vi "ActivateToggleControls (SubVI).vi"(0 "Left refnum":refnum<vi>, 1 "Current stage position [mm]":cluster{"X":dbl, "Y":dbl, "Z":dbl}, 5 "Right refnum":refnum<vi>, 7 "Forward refnum":refnum<vi>, 9 "Backward refnum":refnum<vi>, 11 "error in (no error)":errorcluster, 12 "Jog step size":T1) -> (15 "error out":errorcluster)   [LabVIEW 2016]
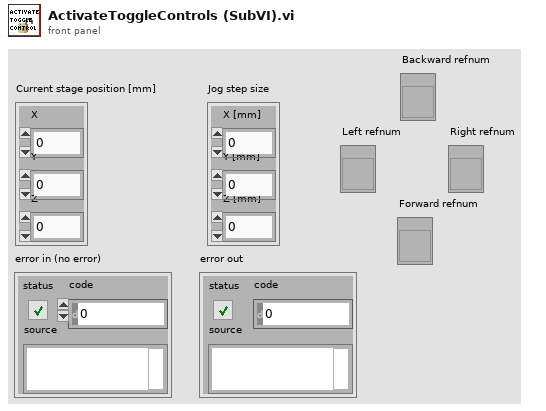
[diagram p1: front panel]
types:
  T1 = cluster{"X [mm]":dbl, "Y [mm]":dbl, "Z [mm]":dbl}
  T2 = enum8{"Enabled", "Disabled", "Disabled and Grayed Out"}
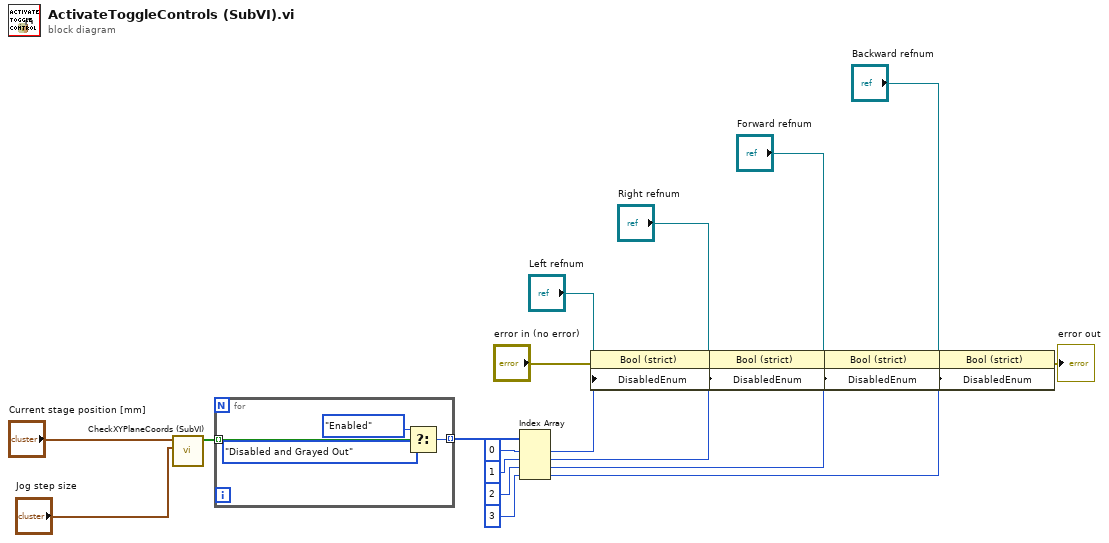
[diagram p0: block diagram]
diagram:
  n1 = call "CheckXYPlaneCoords (SubVI).vi"("Jog Distance"="Jog step size", "Go to Coordinates"="Current stage position [mm]") -> ("Pass record"=w5:bool[])  [unwired: 9 in]
  n2 = for {
    tunnel: w5 -> [w25] mode=indexing
    tunnel: [w22] -> w6 mode=indexing
    n3 = Select(t=T2."Enabled" ("Disabled"), s=w25, f=T2."Disabled and Grayed Out" ("Disabled")) -> (s? t:f=w22:T2)
  }
  n4 = Index Array(array=w6, index #1=0 ("index"), index #2=1 ("index"), index #3=2 ("index"), index #4=3 ("index")) -> (element #1=w11:T2, element #2=w12:T2, element #3=w14:T2, element #4=w16:T2)
  n5 = property on="Property Node" class="Bool (strict)"(reference="Left refnum", error in="error in (no error)", "DisabledEnum"=w11) -> (error out=w13:errorcluster)  [unwired: 1 out]
  n6 = property on="Property Node" class="Bool (strict)"(reference="Right refnum", error in=w13, "DisabledEnum"=w12) -> (error out=w15:errorcluster)  [unwired: 1 out]
  n7 = property on="Property Node" class="Bool (strict)"(reference="Forward refnum", error in=w15, "DisabledEnum"=w14) -> (error out=w17:errorcluster)  [unwired: 1 out]
  n8 = property on="Property Node" class="Bool (strict)"(reference="Backward refnum", error in=w17, "DisabledEnum"=w16) -> (error out=→"error out":errorcluster)  [unwired: 1 out]
